vi "Configure Return Delay.vi"(8 "error in (no error)":errorcluster, 9 "Return Delay (500 microseconds)":sgl=500.0, 10 "Motor ID (0)":u8, 11 "VISA resource name":refnum<visa-resource-name>) -> (0 "error out":errorcluster, 3 "VISA resource name out":refnum<visa-resource-name>)   [LabVIEW 2016, in "Dynamixel Motor.lvlib"]
doc: "Sets the return delay time for the motor."
uses:
  Dynamixel Motor.lvlib
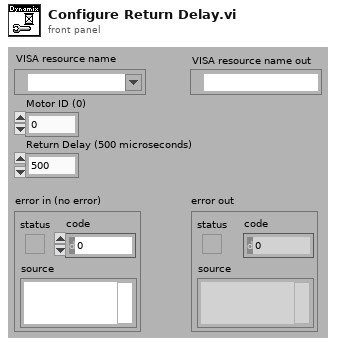
[diagram p1: front panel]
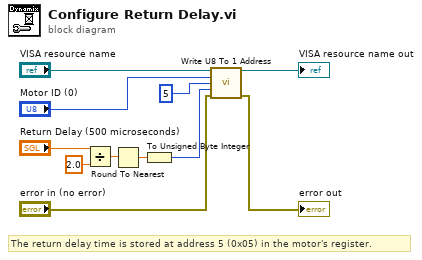
[diagram p0: block diagram]
diagram:
  # "The return delay time is stored at address 5 (0x05) in the motor's register."
  n1 = Divide(x="Return Delay (500 microseconds)", y=sgl 2.0) -> (x/y=w5:sgl)
  n2 = Round To Nearest(number=w5) -> (nearest integer value=w4:sgl)
  n3 = To Unsigned Byte Integer(number=w4) -> (unsigned 8bit integer=w3:u8)
  n4 = call "Write U8 To 1 Address.vi"("VISA resource name"="VISA resource name", "Motor ID (0)"="Motor ID (0)", "Address number (0)"=u8 5 ("Address"), "Parameter (0)"=w3, "error in (no error)"="error in (no error)") -> ("VISA resource name out"=→"VISA resource name out":refnum<visa-resource-name>, "error out"=→"error out":errorcluster)  [unwired: 9 in]
